vi "SetLibraryIcon_FromPath.vi"(8 "error in (no error)":errorcluster, 10 "Icon":refnum<class "Icon.lvclass">, 11 "LibraryPath":path) -> (0 "error out":errorcluster)   [LabVIEW 2014, in "ClassIconTools.lvlib"]
uses:
  <vilib>/LabVIEW Icon API/lv_icon/Classes/Icon/Icon.lvclass
  ClassIconTools.lvlib
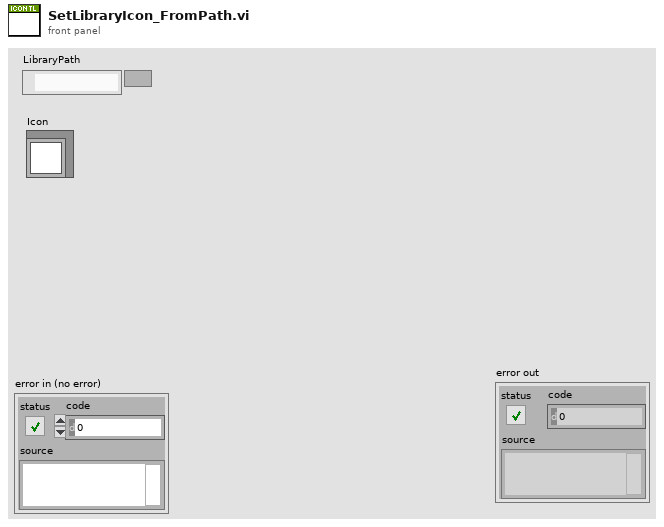
[diagram p1: front panel]
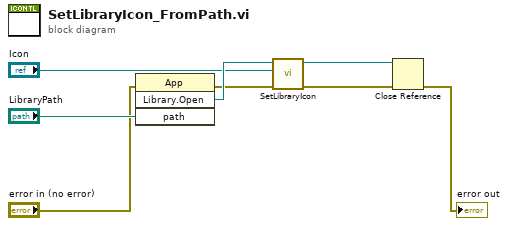
[diagram p0: block diagram]
diagram:
  n1 = invoke class="App" method="Library.Open"(error in="error in (no error)", "path"="LibraryPath") -> (error out=w4:errorcluster, "Open Library"=w6:refnum<vi>)  [unwired: 2 in, 2 out]
  n2 = call "SetLibraryIcon.vi"("error in (no error)"=w4, "Icon"="Icon", "Library"=w6) -> ("error out"=w2:errorcluster, "Library out"=w1:refnum<vi>)  [unwired: 7 in]
  n3 = Close Reference(reference=w1, error in (no error)=w2) -> (error out=→"error out":errorcluster)
